vi "put_element_by_name.vi"(8 "error in (no error)":errorcluster, 9 "value":variant, 10 "name":string, 11 "dataType in":variant) -> (0 "error out":errorcluster, 3 "data out":variant)   [LabVIEW 2015, in "BSON_convertors_Library.lvlib"]
uses:
  BSON_convertors_Library.lvlib
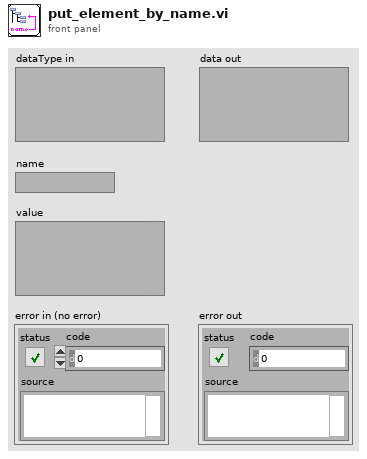
[diagram p1: front panel]
types:
  T1 = typedef "Type Descriptor Enumeration__ogtk.ctl" = enum8{"<Null>", "I8", "I16", "I32", "I64", "U8", "U16", "U32", "U64", "SGL", "DBL", "EXT", "CSG", "CDB", "CXT", "0x0F", "0x10", "0x11", "0x12", "0x13", "0x14", "Enum U8", "Enum U16", "Enum U32", "Enum U64", "SGL PQ", "DBL PQ", "EXT PQ", "CSG PQ", "CDB PQ", "CXT PQ", "0x1F", "0x20", "Boolean", "0x22", "0x23", "0x24", "0x25", "0x26", "0x27", "0x28", "0x29", "0x2A", "0x2B", "0x2C", "0x2D", "0x2E", "0x2F", "String", "0x31", "Path", "Pict", "0x34", "0x35", "0x36", "DAQ", "0x38", "0x39", "0x3A", "0x3B", "0x3C", "0x3D", "0x3E", "0x3F", "Array", "0x41", "0x42", "0x43", "0x44", "0x45", "0x46", "0x47", "0x48", "0x49", "0x4A", "0x4B", "0x4C", "0x4D", "0x4E", "0x4F", "Cluster", "0x51", "0x52", "Variant", "Waveform", "0x55", "0x56", "0x57", "0x58", "0x59", "0x5A", "0x5B", "0x5C", "0x5D", "0x5E", "0x5F", "0x60", "0x61", "0x62", "0x63", "0x64", "0x65", "0x66", "0x67", "0x68", "0x69", "0x6A", "0x6B", "0x6C", "0x6D", "0x6E", "0x6F", "Refnum"}
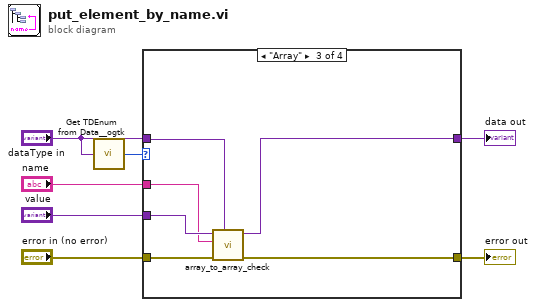
[diagram p0: block diagram]
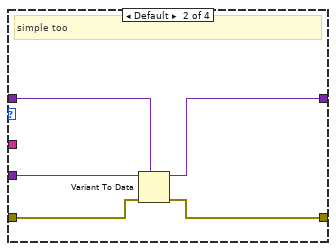
[diagram p3: hidden frame]
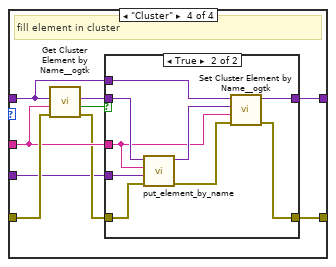
[diagram p4: hidden frame]
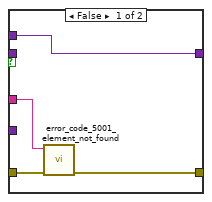
[diagram p5: hidden frame]
diagram:
  n1 = call <userlib>:"Get TDEnum from Data__ogtk.vi"("Data"="dataType in") -> ("Type Descriptor Enumeration"=w1:T1)  [unwired: 4 in]
  n2 = case shown="\"Array\"" w1 {
    tunnel: "dataType in" -> [w9 w12 w18 w22]
    tunnel: [w9 w11 w16 w23] -> w3
    tunnel: "value" -> [_ w14 w20 w21]
    tunnel: "error in (no error)" -> [w8 w13 w19 w29]
    tunnel: [w8 w10 w15 w25] -> w6
    tunnel: "name" -> [_ _ w17 w27]
    frame "<Null>" {
      # "error?\nor not?"
    }
    frame Default {
      # "simple too"
      n3 = Variant To Data(error in=w13, type=w12, Variant=w14) -> (data=w11:variant, error out=w10:errorcluster)
    }
    frame "Array" {
      n4 = call "array_to_array_check.vi"("dataType"=w18, "error in (no error)"=w19, "name"=w17, "value in"=w20) -> ("error out"=w15:errorcluster, "value out"=w16:variant)  [unwired: 6 in]
    }
    frame "Cluster" {
      # "fill element in cluster"
      n5 = call <userlib>:"Get Cluster Element by Name__ogtk.vi"("error in (no error)"=w29, "Element Name"=w27, "Cluster"=w22) -> ("error out"=w26:errorcluster, "found?"=w28:bool, "VElement"=w24:variant)  [unwired: 6 in]
      n6 = case shown="True" w28 {
        tunnel: w27 -> [w33 w34]
        tunnel: w26 -> [w32 w38]
        tunnel: [w31 w40] -> w25
        tunnel: w24 -> [_ w36]
        tunnel: [w30 w41] -> w23
        tunnel: w22 -> [w30 w42]
        tunnel: w21 -> [_ w35]
        frame False {
          n7 = call "error_code_5001_element_not_found.vi"("error in (no error)"=w32, "name"=w33) -> ("error out"=w31:errorcluster)  [unwired: 9 in]
        }
        frame True {
          n8 = call "put_element_by_name.vi"("error in (no error)"=w38, "value"=w35, "name"=w34, "dataType in"=w36) -> ("error out"=w37:errorcluster, "data out"=w39:variant)  [unwired: 6 in]
          n9 = call <userlib>:"Set Cluster Element by Name__ogtk.vi"("error in (no error)"=w37, "Element Name (\"\": New Element Data Name)"=w34, "New Element Value"=w39, "Cluster"=w42) -> ("error out"=w40:errorcluster, "VCluster out"=w41:variant)  [unwired: 5 in, 1 out]
        }
      }
    }
  }
  "error out" <- w6
  "data out" <- w3
